vi "Report File Open.vi"(8 "error in (no error)":errorcluster, 10 "Path":path, 11 "Report File in":refnum<class "Report File.lvclass">) -> (0 "error out":errorcluster, 3 "Report File out":refnum<class "Report File.lvclass">)   [LabVIEW 2018, in "Report File.lvclass"]
uses:
  Report File.lvclass
  Report File.lvclass/Report File.ctl
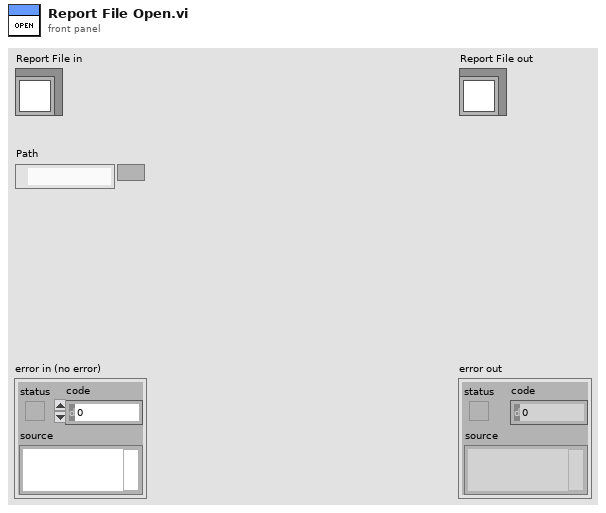
[diagram p1: front panel]
types:
  T1 = enum16{"open", "replace", "create", "open or create", "replace or create", "replace or create with confirmation"}
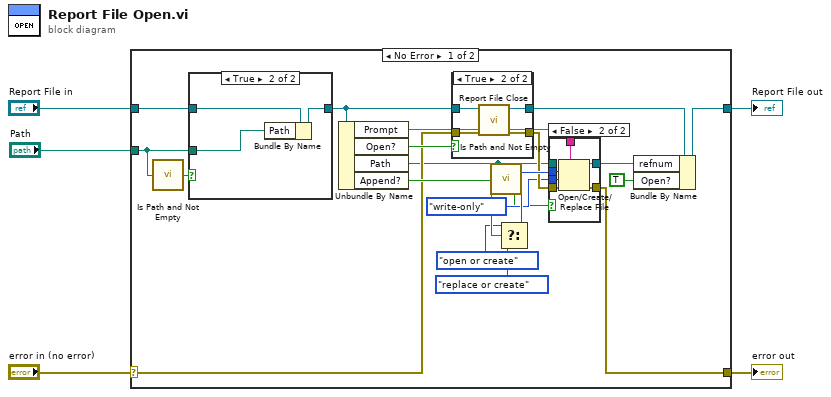
[diagram p0: block diagram]
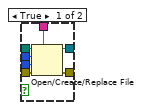
[diagram p2: hidden frame]
diagram:
  n1 = case shown="No Error" "error in (no error)" {
    selector: "error in (no error)" -> [w11 w50]
    tunnel: [w21 w50] -> w4
    tunnel: [w22 w49] -> w2
    tunnel: "Report File in" -> [w23 w49]
    tunnel: "Path" -> [w24 _]
    frame No Error {
      n2 = call <vilib>:"Is Path and Not Empty.vi"("path"=w24) -> ("Is Path and Not Empty?"=w25:bool)  [unwired: 4 in]
      n3 = case shown="True" w25 {
        tunnel: w24 -> [_ w47]
        tunnel: w23 -> [w45 w48]
        tunnel: [w45 w46] -> w13
        frame False {
        }
        frame True {
          n4 = Bundle By Name(cluster=w48, "Path"=w47) -> (w46:refnum<class "Report File.lvclass">)
        }
      }
      n5 = Unbundle By Name(w13) -> ("Prompt"=w8:string, "Open?"=w14:bool, "Path"=w7:path, "Append?"=w20:bool)
      n6 = case shown="True" w14 {
        tunnel: w13 -> [w40 w44]
        tunnel: [w40 w43] -> w12
        tunnel: w11 -> [w39 w42]
        tunnel: [w39 w41] -> w10
        frame False {
        }
        frame True {
          n7 = call-dynamic "Report File Close.vi"("error in (no error)"=w42, "Report File in"=w44) -> ("error out"=w41:errorcluster, "Report File out"=w43:refnum<class "Report File.lvclass">)  [unwired: 8 in]
        }
      }
      n8 = call <vilib>:"Is Path and Not Empty.vi"("path"=w7) -> ("Is Path and Not Empty?"=w6:bool)  [unwired: 4 in]
      n9 = Select(t=T1."open or create" ("operation (0:open)"), s=w20, f=T1."replace or create" ("operation (0:open)")) -> (s? t:f=w19:T1)
      n10 = case shown="False" w6 {
        tunnel: [w32 w38] -> w21
        tunnel: w7 -> [w31 _]
        tunnel: w19 -> [w30 w37]
        tunnel: [w29 w36] -> w16
        tunnel: w10 -> [w28 w35]
        tunnel: enum16{"read/write", "read-only", "write-only"}."write-only" ("access (0:read/write)") -> [w27 w34]
        tunnel: w8 -> [w26 w33]
        frame True {
          n11 = Open/Create/Replace File(file path (use dialog)=w31, error in=w28, prompt=w26, operation (0:open)=w30, access (0:read/write)=w27) -> (refnum out=w29:refnum<file>, error out=w32:errorcluster)  [unwired: 1 in, 1 out]
        }
        frame False {
          n12 = Open/Create/Replace File(error in=w35, prompt=w33, operation (0:open)=w37, access (0:read/write)=w34) -> (refnum out=w36:refnum<file>, error out=w38:errorcluster)  [unwired: 2 in, 1 out]
        }
      }
      n13 = Bundle By Name(cluster=w12, "refnum"=w16, "Open?"=TRUE) -> (w22:refnum<class "Report File.lvclass">)
    }
    frame Error {
    }
  }
  "error out" <- w4
  "Report File out" <- w2
